vi "mkGetSetCamera.vi"() -> ()   [LabVIEW 2011]
uses:
  CameraConfig.ctl
panel:
  in  "Camera settings (in)":T1={"Frame rate (Hz)"=10, "Gain [1-4]"=1024.0, "Offset"=75, "Exposure time"=50, "Mode"=1000, "ROIs"=[], "ROI Size"={"X"=0, "Y"=0}, "Number of buffers"=40} {"Exposure time" min=50}
  in  "IMAQ Refnum in":refnum<k11>
  # "us"
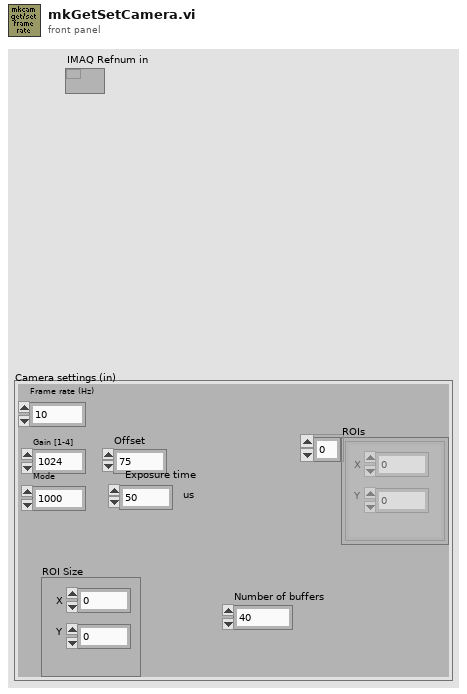
[diagram p1: front panel]
types:
  T1 = typedef "CameraConfig.ctl" = cluster{"Frame rate (Hz)":u32, "Gain [1-4]":sgl, "Offset":i16, "Exposure time":i32, "Mode":i16, "ROIs":cluster{"X":i32, "Y":i32}[], "ROI Size":cluster{"X":i32, "Y":i32}, "Number of buffers":i32}
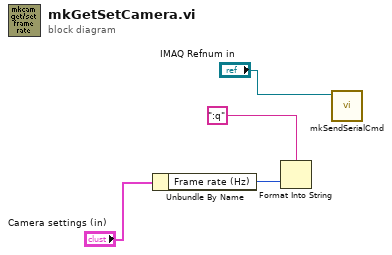
[diagram p0: block diagram]
diagram:
  n1 = Unbundle By Name("Camera settings (in)") -> ("Frame rate (Hz)"=w1:u32)
  n2 = Format Into String(format string=":q" ("String"), w1) -> ()  [unwired: 2 in, 2 out]
  n3 = call "mkSendSerialCmd.vi"("IMAQ Refnum in"="IMAQ Refnum in") -> ()  [unwired: 7 in, 4 out]
